vi "Log Data.vi"(8 "error in (no error)":errorcluster, 10 "Data Queue":refnum<queue>, 11 "Logging Configuration":T1={"Log File Base Path"=path "", "NbrIma"=1} {"NbrIma" min=1 step=1}) -> (0 "error out":errorcluster)   [LabVIEW 2020, in "Logging.lvlib"]
doc: "This VI uses the TDMS Write function to write data to a TDMS file."
uses:
  Logging.lvlib
  Logging Configuration.ctl
  SETTING/data_Queue.ctl
  FITS/BigDataFits.ctl
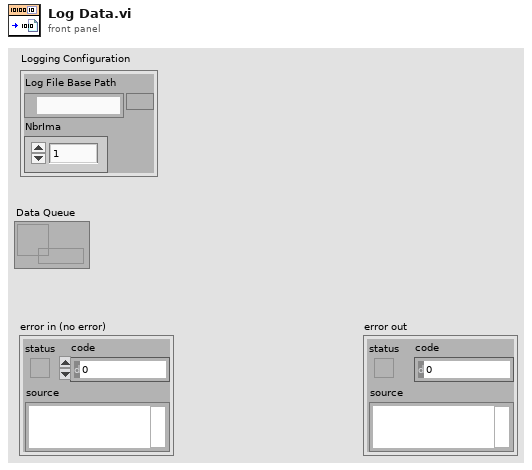
[diagram p1: front panel]
types:
  T1 = typedef "Logging.lvlib/Logging Configuration.ctl" = cluster{"Log File Base Path":path, "NbrIma":i32}
  T2 = typedef "BigDataFits.ctl" = enum16{"Init", "WritHeader", "WritData", "Close"}
  T3 = typedef "data_Queue.ctl" = cluster{"tabIma":u16[][], "tabCdG":sgl[], "vectCom":sgl[]}
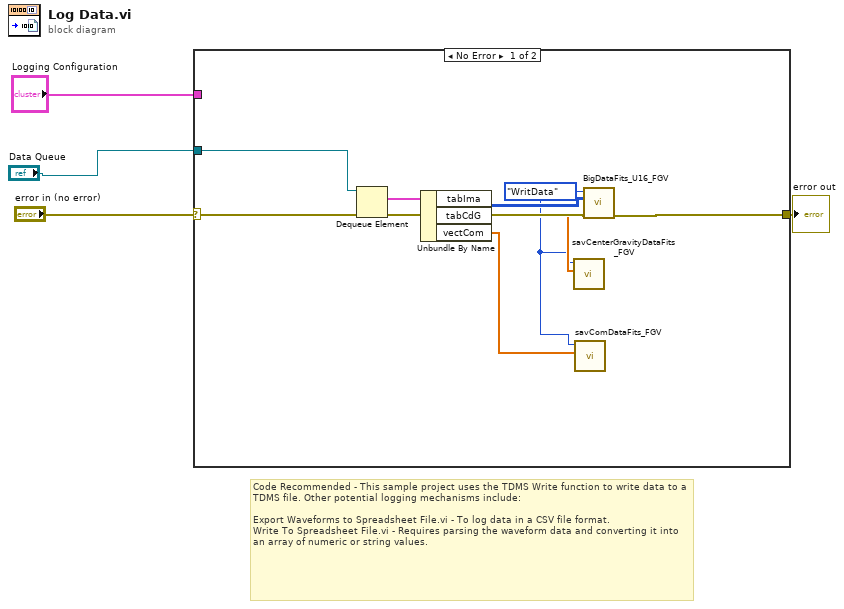
[diagram p0: block diagram]
diagram:
  # "Code Recommended - This sample project uses the TDMS Write function to write data to a TDMS file. Other potential logging mechanisms include:\n\nExport Waveforms to Spreadsheet File.vi - To log data in a CSV file format.\nWrite To Spreadsheet File.vi - Requires parsing the waveform data and converting it into an array of numeric or string values."
  n1 = case shown="No Error" "error in (no error)" {
    selector: "error in (no error)" -> [w13 w14]
    tunnel: "Logging Configuration" -> [_ _]
    tunnel: "Data Queue" -> [w12 _]
    tunnel: [w11 w14] -> w3
    frame No Error {
      w5 = BigDataFits."WritData" ("Énum")
      n2 = Dequeue Element(queue=w12, error in (no error)=w13) -> (element=w9:T3, error out=w10:errorcluster)  [unwired: 1 in, 2 out]
      n3 = Unbundle By Name(w9) -> ("tabIma"=w8:u16[][], "tabCdG"=w6:sgl[], "vectCom"=w7:sgl[])
      n4 = call "savCenterGravityDataFits_FGV.vi"("SGL 32 bits"=w6, "Énum"=w5) -> ()  [unwired: 9 in, 1 out]
      n5 = call "savComDataFits_FGV.vi"("SGL 32 bits"=w7, "Énum"=w5) -> ()  [unwired: 9 in, 1 out]
      n6 = call "BigDataFits_U16_FGV.vi"("InError"=w10, "entier 16 bits"=w8, "Énum"=w5) -> ("sortie d'erreur"=w11:errorcluster)  [unwired: 8 in]
    }
    frame Error {
    }
  }
  "error out" <- w3
